vi "nejistota_A.vi"(10 "No to avg":i32, 11 "Array":dbl[](array[numeric])) -> (2 "nejistota_A":dbl, 3 "mean":dbl)   [LabVIEW 2022 SP3]
uses:
  <vilib>/Analysis/NI_AALBase.lvlib
  <vilib>/Analysis/NI_AALBLAS.lvlib
  <vilib>/Analysis/baseanly.llb/Mean (DBL).vi
  <vilib>/Analysis/BLAS.llb/dasum - Absolute Values Sum (DBL).vi
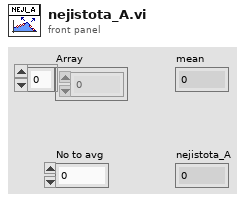
[diagram p1: front panel]
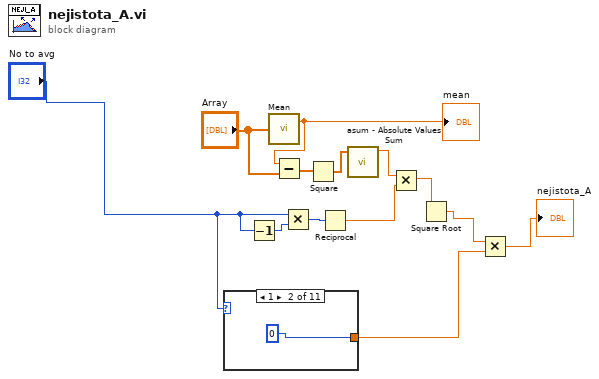
[diagram p0: block diagram]
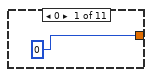
[diagram p2: hidden frame]
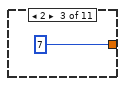
[diagram p3: hidden frame]
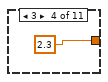
[diagram p4: hidden frame]
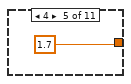
[diagram p5: hidden frame]
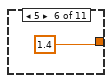
[diagram p6: hidden frame]
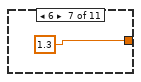
[diagram p7: hidden frame]
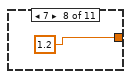
[diagram p8: hidden frame]
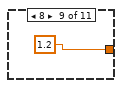
[diagram p9: hidden frame]
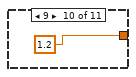
[diagram p10: hidden frame]
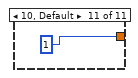
[diagram p11: hidden frame]
diagram:
  n1 = case shown="1" "No to avg" {
    tunnel: [0 0 7 2.3 1.7 1.4 1.3 1.2 1.2 1.2 1] -> w3
    frame 0 {
    }
    frame 1 {
    }
    frame 2 {
    }
    frame 3 {
    }
    frame 4 {
    }
    frame 5 {
    }
    frame 6 {
    }
    frame 7 {
    }
    frame 8 {
    }
    frame 9 {
    }
    frame 10, Default {
    }
  }
  n2 = Decrement(x="No to avg") -> (x-1=w9:i32)
  n3 = call-poly <vilib>:"Mean.vi"("X"="Array") -> ("mean"=w5:dbl)  [unwired: 1 out]
  "mean" <- w5
  n4 = Subtract(x=w5, y="Array") -> (x-y=w7:dbl[])
  n5 = Multiply(x="No to avg", y=w9) -> (x*y=w10:i32)
  n6 = Square(x=w7) -> (x^2=w8:dbl[])
  n7 = Reciprocal(x=w10) -> (1/x=w12:dbl)
  n8 = call-poly <vilib>:"asum - Absolute Values Sum.vi"("x"=w8) -> ("dasum"=w11:dbl)  [unwired: 9 in, 1 out]
  n9 = Multiply(x=w11, y=w12) -> (x*y=w13:dbl)
  n10 = Square Root(x=w13) -> (sqrt(x)=w2:dbl)
  n11 = Multiply(x=w2, y=w3) -> (x*y=→"nejistota_A":dbl)
